vi "Double FFT Measurement test.vi"   [LabVIEW 2014]
uses:
  <vilib>/Platform/TimedLoop/XDataNode/timing_clust.ctl
  <vilib>/Platform/TimedLoop/XDataNode/nitl_modes.ctl
  <vilib>/Platform/TimedLoop/XDataNode/wakeup.ctl
  <vilib>/rvi/Analysis/measure/FFT/simModelSupport/niFPGA FFT Streaming Sim Properties.ctl
  <vilib>/rvi/Analysis/measure/FFT/simModelSupport/niFPGA FFT Sim Stream Group Properties.ctl
  <vilib>/rvi/Analysis/measure/FFT/simModelSupport/niFPGA FFT Sim Types.ctl
  <vilib>/rvi/Analysis/measure/FFT/simModelSupport/niFpgaFFTSimArithmeticProperties.ctl
  <vilib>/rvi/Analysis/measure/FFT/simModelSupport/niFpgaFFTSimDfxp.ctl
  <vilib>/fxp/LVFixedPointQuantizationPolicyTypeDef.ctl
  <vilib>/rvi/Analysis/measure/FFT/XNode/niFpgaFFTButterflyDelays.ctl
  <vilib>/rvi/Emulation/niFpgaSctlEmulationGetInTimedLoop.vi
  <vilib>/rvi/Emulation/niFpgaEmulationReportErrorSimple.vi
  <vilib>/rvi/Emulation/niFpgaGetClockAttributes.vi
  <vilib>/rvi/Emulation/niFpgaCriticalErrorInLSC.vi
  <vilib>/rvi/Emulation/niFpgaEmulationIsFPGAContextNoSignature.vi
  <vilib>/rvi/errors/niFpgaSetErrorForExecOnDevCompSimple.vi
  <vilib>/rvi/eio/common/nirviEmuReportErrorAndStop.vi
  <vilib>/rvi/DataTransferAndStorage/Container/Common/niFpgaContainerGetUniqueNameForEmu.vi
  <vilib>/rvi/FIFO/Fifo_Resource/nirvififoEmulationSetSize.vi
  <vilib>/rvi/FIFO/Fifo_Resource/nirviFifoEmulationQueueMgr.vi
  <instcachedir>/0/nirviFifoEmulationQueueMgr_E5CAEC123FF24DC58D834DCA3CDAA9B5.lvgen/nirviFifoEmulationQueueMgr_E5CAEC123FF24DC58D834DCA3CDAA9B5_010.vi
  <vilib>/rvi/FIFO/Fifo_Resource/nirvififoEmulationCreateLock.vi
  <vilib>/rvi/Emulation/niFpgaProcessEmulError.vi
  <vilib>/rvi/FIFO/Fifo_Resource/nirvififoEmulationObtainLock.vi
  <vilib>/rvi/FIFO/Fifo_Resource/nirvififoEmulationReleaseLock.vi
  <vilib>/rvi/occurrence/nirviWaitOnOccurrenceBase.vi
  <vilib>/rvi/errors/nirviReportUnexpectedCaseInternalError.vi
  <vilib>/rvi/errors/nirviReportUnexpectedCaseInternalError (U32).vi
  <vilib>/rvi/FIFO/Fifo_Resource/nirvififoEmulationDetermineInputValidOut.vi
  <vilib>/rvi/Memory/Memory_Emulation/nirvimemoryFastEmulation.vi
  <vilib>/rvi/Memory/Memory_Emulation/nirvimemoryEmulation.vi
  <vilib>/rvi/interface/RandomDataEmulation/niFpgaRandomDataHandleErrors.vi
  <vilib>/rvi/Analysis/measure/FFT/simModelSupport/niFpgaFFTSimModelStreamingCore.vi
  <vilib>/rvi/eio/common/nirviEmuTemplateMethod_errors.vi
  <vilib>/Platform/TimedLoop/XDataNode/XDataNode.xnode
  <vilib>/rvi/DataTransferAndStorage/Container/XNode/niFpgaContainer.xnode
  <vilib>/rvi/FIFO/Fifo_Resource/nirvififoEmulationRead.vi
  <vilib>/rvi/FIFO/Fifo_Resource/nirvififoEmulationWrite.vi
  <vilib>/rvi/interface/RandomDataEmulation/nirviRandomDataFpgaReadWriteTemplate.vi
  <vilib>/rvi/Analysis/measure/FFT/XNode/niFpgaFFT.xnode
  <vilib>/eio/EIOMethodNode/EIOMethodNode.xnode
  <vilib>/Platform/TimedLoop/XDataNode/XDNodeRunTimeDep.lvlib
types:
  T1 = typedef "XDNodeRunTimeDep.lvlib/timing_clust.ctl" = cluster{"Expected End [f-1]":u64, "Actual End [f-1]":u64, "Finished Late? [f-1]":bool, "Expected End [i-1]":u64, "Actual End [i-1]":u64, "Finished Late? [i-1]":bool, "Expected Start [i]":u64, "Actual Start [i]":u64, "Expected Start [f]":u64, "Actual Start [f]":u64, "Source Name":string, "Structure Name":string, "Period":i64, "Deadline":i64, "Offset":i64, "Start":i64, "Priority":i32, "Timeout":i32, "Mode":T2, "Wakeup Reason":T3, "Error":errorcluster, "Source Type":string, "Secondary Source Type":string, "Global End Time":u64, "Global Start Time":u64, "Frame Duration":u64, "Iteration Duration":u64, "Assigned CPU":i32, "I/O Scan Engine Mode":u32}
  T2 = typedef "XDNodeRunTimeDep.lvlib/nitl_modes.ctl" = enum32{"No Change", "Process missed periods, maintain original phase", "Discard missed periods, maintain original phase", "Process missed periods, ignore original phase", "Discard missed periods, ignore original phase"}
  T3 = typedef "XDNodeRunTimeDep.lvlib/wakeup.ctl" = enum32{"Normal", "Aborted", "Asynchronous wakeup", "Timing source error", "Timed loop error", "Timeout"}
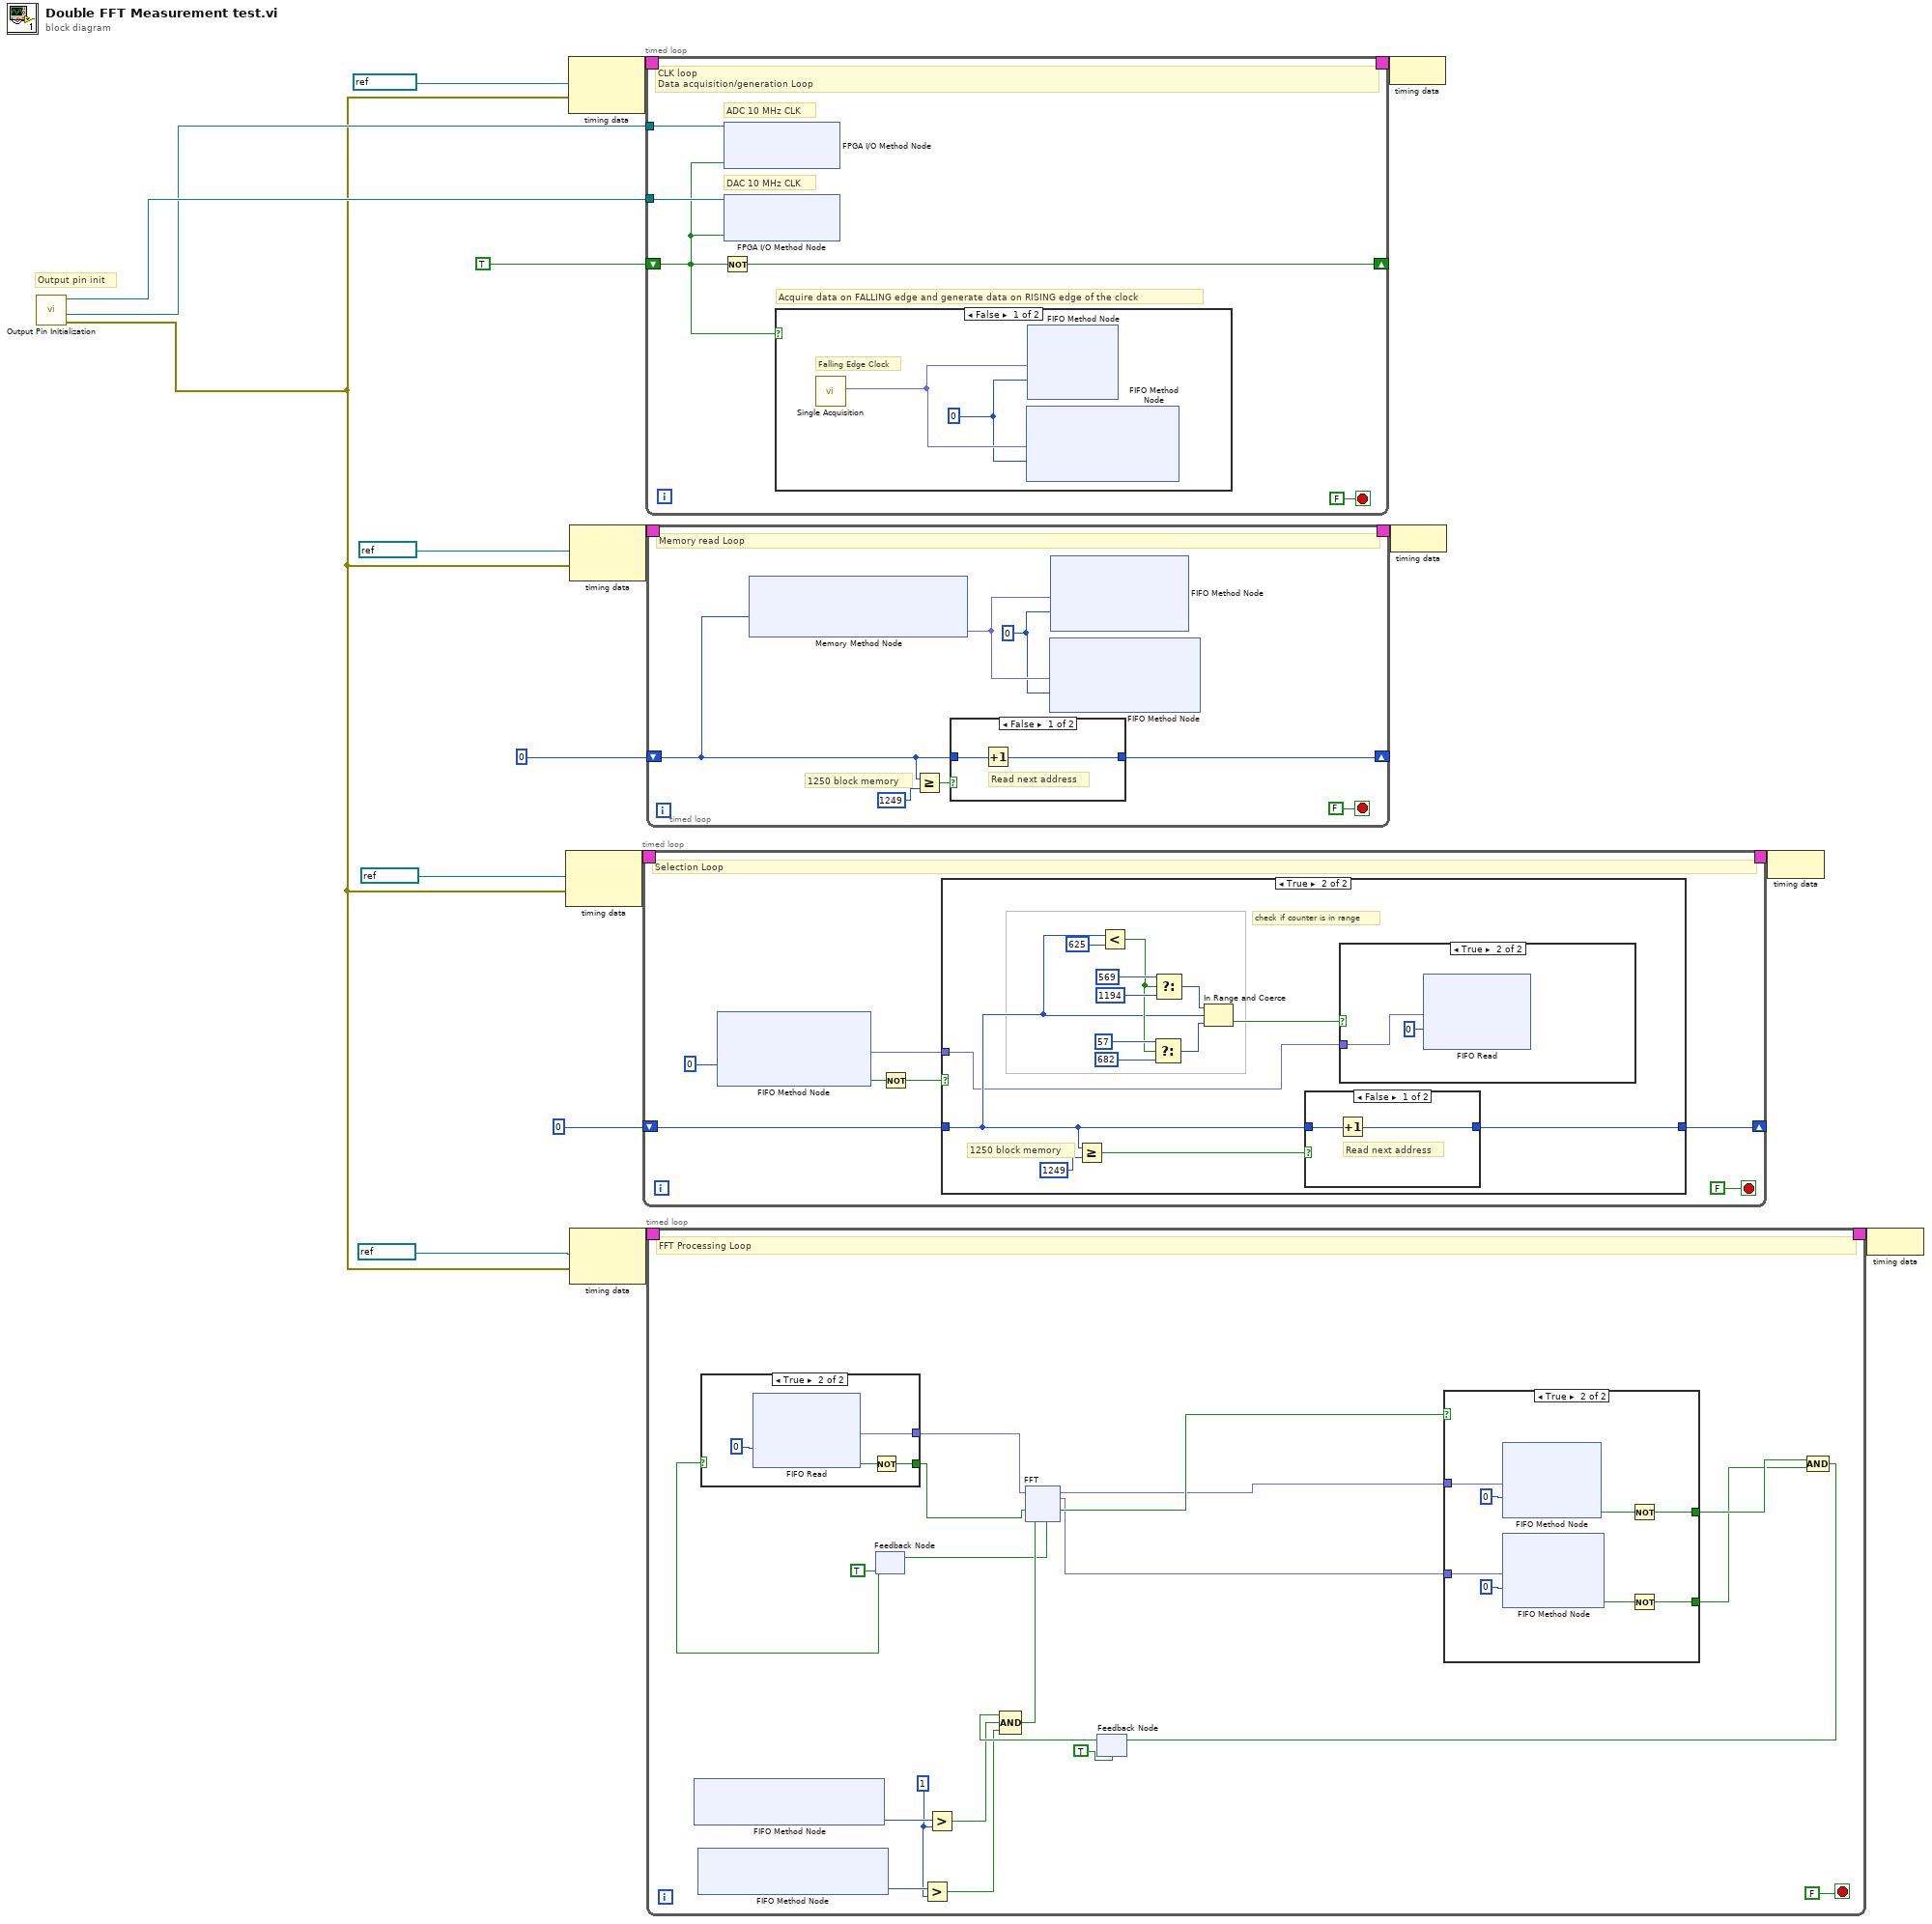
[diagram p0: block diagram]
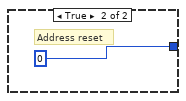
[diagram p4: hidden frame]
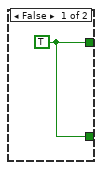
[diagram p5: hidden frame]
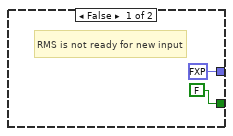
[diagram p6: hidden frame]
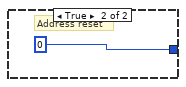
[diagram p7: hidden frame]
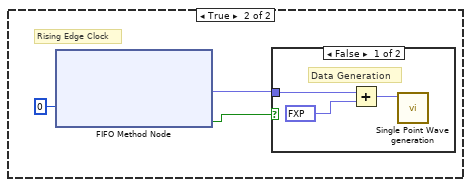
[diagram p8: hidden frame]
diagram:
  # "Output pin init"
  n1 = call "Output Pin Initialization.vi"() -> ("error out"=w3:errorcluster, "I/O Out Clock DAC (pin16)"=w6:refnum<k21>, "I/O Out Clock ADC (pin17)"=w7:refnum<k21>)  [unwired: 8 in]
  n2 = node-c288(refnum<k21> "50MHz" ("Source Name"), w3) -> (w5:T1)
  n3 = node-c288(refnum<k21> "100MHz" ("Source Name"), w3) -> (w18:T1)
  n4 = node-c288(refnum<k21> "50MHz" ("Source Name"), w3) -> (w16:T1)
  n5 = node-c288(refnum<k21> "50MHz" ("Source Name"), w3) -> (w14:T1)
  n6 = timed-loop {
    timing: w5 -> [_]
    timing-out: [_] -> w4
    shift-right: [w24] -> _
    shift-left: u32 0 -> [w23]
    stop <- FALSE stop-if-true
    # "Selection Loop"
    n7 = xnode ("FIFO Method Node")("Timeout"=0) -> ("Element"=w20:fxp<+/-,12,12>, "Timed Out?"=w21:bool)  [unwired: 1 in, 1 out]
    n8 = Not(x=w21) -> (.not. x?=w22:bool)
    n9 = case shown="True" w22 {
      tunnel: [w26 w38] -> w24
      tunnel: w23 -> [w26 w29]
      tunnel: w20 -> [_ w27]
      frame False {
      }
      frame True {
        # "check if counter is in range"
        # "1250 block memory"
        n10 = Greater Or Equal?(x=w29, y=u32 1249) -> (x >= y?=w39:bool)
        n11 = Less?(x=w29, y=u32 625) -> (x < y?=w30:bool)
        n12 = Select(t=u32 57 ("lower limit"), s=w30, f=u32 682 ("lower limit")) -> (s? t:f=w32:u32)
        n13 = Select(t=u32 569 ("upper limit"), s=w30, f=u32 1194 ("upper limit")) -> (s? t:f=w33:u32)
        n14 = In Range and Coerce(upper limit=w33, x=w29, lower limit=w32) -> (In Range?=w28:bool)  [unwired: 1 out]
        n15 = case shown="False" w39 {
          tunnel: w29 -> [w44 _]
          tunnel: [w43 u32 0] -> w38
          frame False {
            # "Read next address"
            n16 = Increment(x=w44) -> (x+1=w43:u32)
          }
          frame True {
            # "Address reset"
          }
        }
        n17 = case shown="True" w28 {
          tunnel: w27 -> [_ w42]
          frame False {
          }
          frame True {
            n18 = xnode ("FIFO Read")("Element"=w42, "Timeout"=0) -> ()  [unwired: 1 in, 2 out]
          }
        }
      }
    }
  }
  n19 = timed-loop {
    timing: w18 -> [_]
    timing-out: [_] -> w17
    shift-right: [w50] -> _
    shift-left: TRUE -> [w48]
    tunnel: w6 -> [w52]
    tunnel: w7 -> [w49]
    stop <- FALSE stop-if-true
    # "DAC 10 MHz CLK"
    # "Acquire data on FALLING edge and generate data on RISING edge of the clock"
    # "ADC 10 MHz CLK"
    # "CLK loop\nData acquisition/generation Loop"
    n20 = Not(x=w48) -> (.not. x?=w50:bool)
    n21 = xnode "FPGA I/O Method Node"("FPGA I/O In"=w52, "Data"=w48) -> ()  [unwired: 1 out]
    n22 = xnode "FPGA I/O Method Node"("FPGA I/O In"=w49, "Data"=w48) -> ()  [unwired: 1 out]
    n23 = case shown="False" w48 {
      frame False {
        w53 = 0 ("Timeout")
        # "Falling Edge Clock"
        n24 = call "Single Acquisition.vi"() -> ("Out"=w54:fxp<+/-,12,12>)  [unwired: 10 in, 1 out]
        n25 = xnode ("FIFO Method Node")("Element"=w54, "Timeout"=w53) -> ()  [unwired: 1 in, 2 out]
        n26 = xnode ("FIFO Method Node")("Element"=w54, "Timeout"=w53) -> ()  [unwired: 1 in, 2 out]
      }
      frame True {
        # "Rising Edge Clock"
        n27 = xnode ("FIFO Method Node")("Timeout"=0) -> ("Element"=w55:fxp<+/-,12,12>, "Timed Out?"=w56:bool)  [unwired: 1 in, 1 out]
        n28 = case shown="False" w56 {
          tunnel: w55 -> [w60 _]
          frame False {
            # "Data Generation"
            n29 = Add(x=w60, y=fxp<+,12,12> 2048.0) -> (x+y=w58:fxp<+/-,14,14>)
            n30 = call "Single Point Wave generation.vi"("Data To Write"=w58) -> ()  [unwired: 10 in, 1 out]
          }
          frame True {
            # "FPGA memory slow"
          }
        }
      }
    }
  }
  n31 = timed-loop {
    timing: w16 -> [_]
    timing-out: [_] -> w15
    shift-right: [w67] -> _
    shift-left: u32 0 -> [w65]
    stop <- FALSE stop-if-true
    w63 = 0 ("Timeout")
    # "1250 block memory"
    # "Memory read Loop"
    n32 = xnode ("Memory Method Node")("Address"=w65) -> ("Data"=w64:fxp<+/-,12,12>)  [unwired: 1 in, 1 out]
    n33 = Greater Or Equal?(x=w65, y=u32 1249) -> (x >= y?=w68:bool)
    n34 = case shown="False" w68 {
      tunnel: w65 -> [w71 _]
      tunnel: [w70 u32 0] -> w67
      frame False {
        # "Read next address"
        n35 = Increment(x=w71) -> (x+1=w70:u32)
      }
      frame True {
        # "Address reset"
      }
    }
    n36 = xnode ("FIFO Method Node")("Element"=w64, "Timeout"=w63) -> ()  [unwired: 1 in, 2 out]
    n37 = xnode ("FIFO Method Node")("Element"=w64, "Timeout"=w63) -> ()  [unwired: 1 in, 2 out]
  }
  n38 = timed-loop {
    timing: w14 -> [_]
    timing-out: [_] -> w13
    stop <- FALSE stop-if-true
    w77 = u32 1 ("y")
    # "FFT Processing Loop"
    n39 = xnode ("FIFO Method Node")() -> ("Number of Elements to Write"=w79:u32)  [unwired: 1 in, 1 out]
    n40 = xnode ("FIFO Method Node")() -> ("Number of Elements to Write"=w78:u32)  [unwired: 1 in, 1 out]
    n41 = feedback #1(TRUE ("ready for input")) -> (w94:bool)
    n42 = case shown="True" w94 {
      tunnel: [FALSE w135] -> w88
      tunnel: [fxp<+/-,12,12> 0.0 ("Element") w132] -> w89
      frame False {
        # "RMS is not ready for new input"
      }
      frame True {
        n43 = xnode ("FIFO Read")("Timeout"=0) -> ("Element"=w132:fxp<+/-,12,12>, "Timed Out?"=w134:bool)  [unwired: 1 in, 1 out]
        n44 = Not(x=w134) -> (.not. x?=w135:bool)
      }
    }
    n45 = Greater?(x=w78, y=w77) -> (0:w75:bool)
    n46 = Greater?(x=w79, y=w77) -> (0:w76:bool)
    n47 = feedback #2(TRUE) -> (w90:bool)
    n48 = Compound Arithmetic op=AND(w90, w76, w75) -> (w87:bool)
    n49 = xnode "FFT"("real data in"=w89, "input valid"=w88, "ready for output"=w87) -> ("ready for input"=w86:bool, "real data out"=w84:fxp<+/-,22,22>, "imaginary data out"=w83:fxp<+/-,22,22>, "output valid"=w85:bool)  [unwired: 2 in, 1 out]
    n50 = feedback-in #1(w86) -> ()
    n51 = case shown="True" w85 {
      tunnel: w84 -> [_ w129]
      tunnel: w83 -> [_ w128]
      tunnel: [w121 w127] -> w82
      tunnel: [w121 w126] -> w81
      frame False {
        w121 = TRUE
      }
      frame True {
        n52 = xnode ("FIFO Method Node")("Element"=w129, "Timeout"=0) -> ("Timed Out?"=w122:bool)  [unwired: 1 in, 1 out]
        n53 = xnode ("FIFO Method Node")("Element"=w128, "Timeout"=0) -> ("Timed Out?"=w123:bool)  [unwired: 1 in, 1 out]
        n54 = Not(x=w122) -> (.not. x?=w127:bool)
        n55 = Not(x=w123) -> (.not. x?=w126:bool)
      }
    }
    n56 = Compound Arithmetic op=AND(w82, w81) -> (w80:bool)
    n57 = feedback-in #2(w80) -> ()
  }
  n58 = node-c288(w17) -> ()
  n59 = node-c288(w15) -> ()
  n60 = node-c288(w4) -> ()
  n61 = node-c288(w13) -> ()
